vi "Find_Names_Containing.vi"(2 "Ch names":string[](array[string]), 3 "String to match":string) -> (0 "Indicies":i32[](array[numeric]), 1 "Matched Names":string[](array[string]))   [LabVIEW 2010]
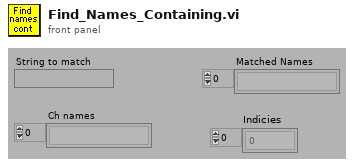
[diagram p1: front panel]
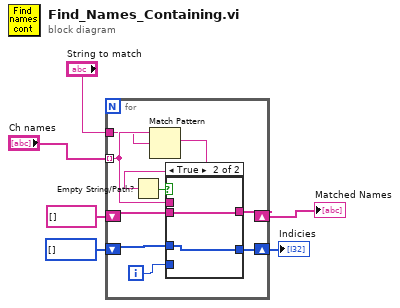
[diagram p0: block diagram]
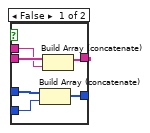
[diagram p2: hidden frame]
diagram:
  n1 = for {
    tunnel: "Ch names" -> [w12] mode=indexing
    shift-right: [w11] -> w5
    shift-left: string[] [] -> [w13]
    tunnel: "String to match" -> [w10]
    shift-right: [w7] -> w1
    shift-left: i32[] [] -> [w8]
    i -> [w9]
    n2 = Match Pattern(string=w12, regular expression=w10) -> (match substring=w15:string)  [unwired: 4 out]
    n3 = Empty String/Path?(string/path=w15) -> (empty?=w14:bool)
    n4 = case shown="True" w14 {
      tunnel: w13 -> [w21 w23]
      tunnel: w12 -> [w20 _]
      tunnel: [w19 w23] -> w11
      tunnel: w9 -> [w18 _]
      tunnel: w8 -> [w17 w22]
      tunnel: [w16 w22] -> w7
      frame False {
        n5 = Build Array (concatenate)(w17, w18) -> (w16:i32[])
        n6 = Build Array (concatenate)(w21, w20) -> (w19:string[])
      }
      frame True {
      }
    }
  }
  "Matched Names" <- w5
  "Indicies" <- w1
